vi "StartMeasurement.vi"(8 "error in (no error)":errorcluster, 11 "object in":refnum<class "Actor1_GUI_N_4.0.0.lvclass">) -> (0 "error out":errorcluster, 3 "object out":refnum<class "Actor1_GUI_N_4.0.0.lvclass">)   [LabVIEW 2020, in "Actor1_GUI_N_4.0.0.lvlib" / "Actor1_GUI_N_4.0.0.lvclass"]
uses:
  <resource>/Framework/Providers/Open_GDS/ClassProviders/ActorFramework/4.0.0/Actor1_GUI_N_4.0.0/Actor1_GUI_N_4.0.0_class/Actor1_GUI_N_4.0.0.lvclass
  <resource>/Framework/Providers/Open_GDS/ClassProviders/ActorFramework/4.0.0/Actor1_GUI_N_4.0.0/Actor1_GUI_N_4.0.0_class/Actor1_GUI_N_4.0.0.lvclass/Actor1_GUI_N_4.0.0.ctl
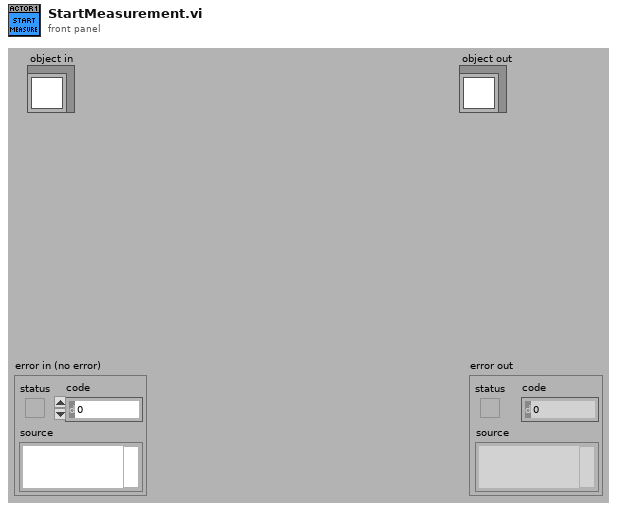
[diagram p1: front panel]
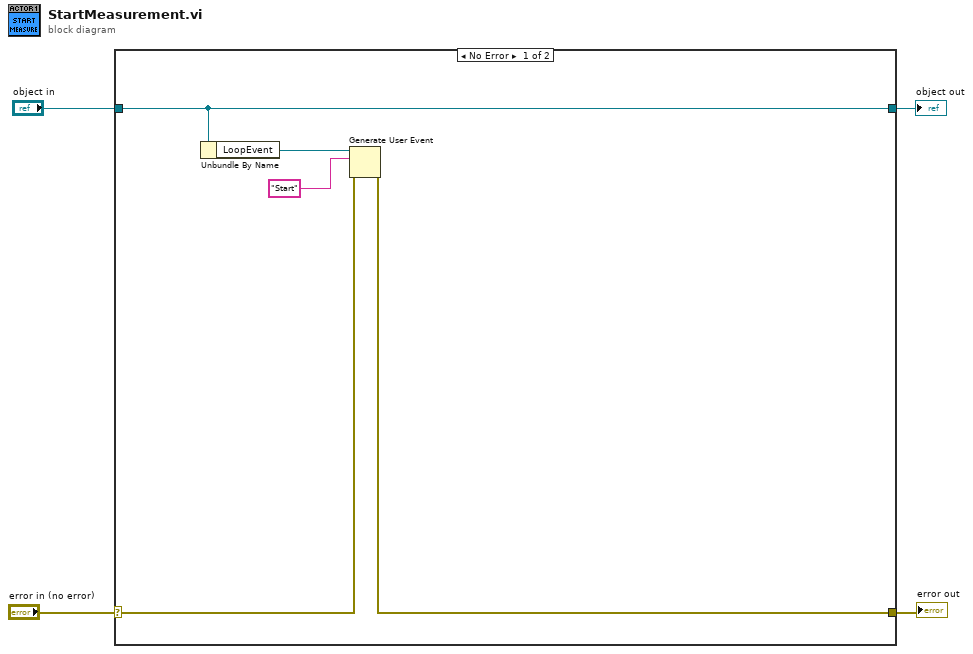
[diagram p0: block diagram]
diagram:
  n1 = case shown="No Error" "error in (no error)" {
    selector: "error in (no error)" -> [w7 w11]
    tunnel: [w6 w11] -> w3
    tunnel: [w9 w10] -> w1
    tunnel: "object in" -> [w9 w10]
    frame No Error {
      n2 = Unbundle By Name(w9) -> ("LoopEvent"=w8:refnum<user-event>)
      n3 = Generate User Event(user event=w8, event data cluster="Start", error in=w7) -> (error out=w6:errorcluster)  [unwired: 1 in, 1 out]
    }
    frame Error {
    }
  }
  "error out" <- w3
  "object out" <- w1
